vi "Parse.vi"(8 "Error In":errorcluster, 11 "object in":refnum<class "2024_2.lvclass">) -> (0 "Error Out":errorcluster, 3 "object out":refnum<class "2024_2.lvclass">)   [LabVIEW 2023, in "2024_2.lvclass"]
uses:
  2024_2.lvclass
  2024_2.lvclass/2024_2.ctl
  <vilib>/Utility/error.llb/Trim Whitespace One-Sided.vi
  <userlib>/_OpenG.lib/string/string.llb/openg_string.lvlib
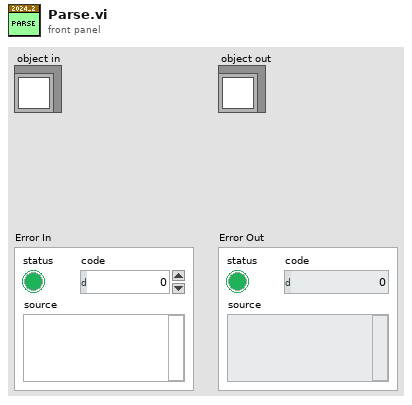
[diagram p1: front panel]
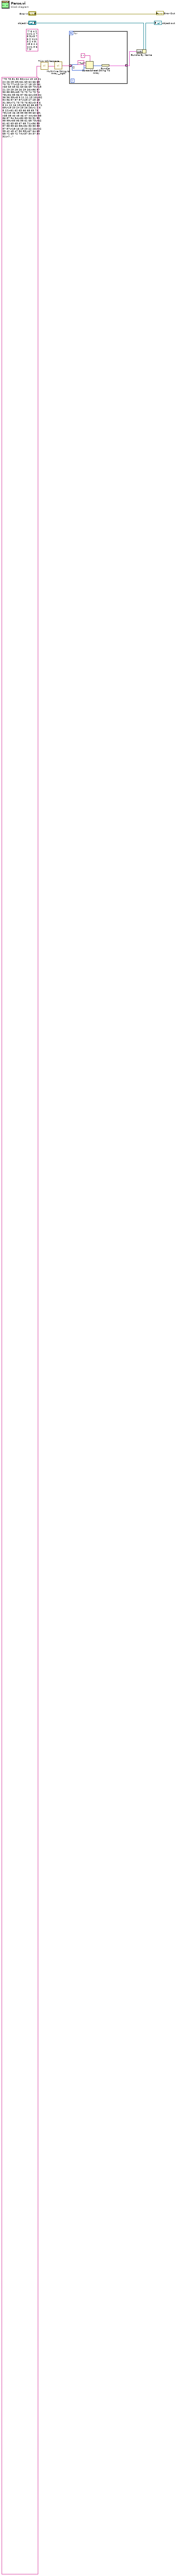
[diagram p0: block diagram]
diagram:
  (unwired) "7 6 4 2 1\n1 2 7 8 9\n9 7 6 2 1\n1 3 2 4 5\n8 6 4 4 1\n1 3 6 7 9" ("PuzzleInput")
  n1 = call <vilib>:"Trim Whitespace.vi"("string"="75 78 81 82 80\n14 15 18 21 24 26 28 28\n61 63 64 66 68 70 73 77\n13 14 17 18 19 26\n60 63 65 62 63 66 69 70\n18 21 23 25 28 26 29 26\n86 87 90 88 88\n69 70 73 74 73 74 78\n54 55 56 57 56 62\n33 34 36 36 39\n8 9 11 11 13 10\n52 54 56 57 57 57\n25 27 28 28 31 35\n71 73 73 76 82\n3 5 6 8 11 12 16 19\n59 62 66 69 71 69\n19 20 24 25 26 26\n1 2 6 8 12\n61 62 63 66 68 69 73 78\n43 46 48 55 58 59 60 63\n35 38 40 45 46 47 44\n84 85 86 87 94 94\n80 83 90 91 93 95 99\n53 56 58 61 68 73\n62 61 62 63 65 67 68 71\n56 55 57 58 59 60 58\n52 50 53 55 57 57\n18 16 19 20 22 26\n42 39 42 45 47 50 55\n67 64 65 68 71 69 72 74\n37 34 37 34 31\n75 72 74 73 75 77 77\n90 88 90 91 90 91 95\n72 70 72 69 70 76\n71 70 71 71 73\n83 80 80 81 80\n68 66 69 72 72 75 75\n45 44 45 48 48 50 54\n64 62 65 65 72\n39 37 39 43 46 48 51 52\n28 27 31 33 32\n25 22 26 29 29\n72 71 72 75 79 82 86\n70 68 71 75 76 78 81 88\n89 87 89 90 96 97\n8 7 9 14 17 16\n31 29 30 37 40 43 45 45\n44 41 43 50 52 53 57\n4 1 2 9 15\n6 6 9 11 12 13 16\n36 36 37 40 43 45 47 46\n88 88 89 91 94 94\n13 13 16 19 21 22 26\n17 17 19 20 21 24 26 31\n21 21 22 21 24\n73 73 71 72 74 77 80 79\n31 31 33 34 37 36 36\n21 21 20 23 27\n31 31 29 31 37\n55 55 58 60 60 63 64\n28 28 31 31 29\n69 69 70 73 74 74 74\n12 12 15 17 18 18 19 23\n5 5 5 6 13\n61 61 63 67 68\n37 37 39 42 43 47 46\n76 76 79 82 86 86\n43 43 47 50 53 55 56 60\n51 51 52 55 59 60 67\n75 75 78 81 88 90 92\n53 53 55 57 59 61 68 67\n86 86 87 88 94 94\n60 60 62 64 67 74 78\n71 71 74 81 83 86 93\n22 26 29 30 31 32 34 36\n47 51 52 55 57 55\n39 43 45 46 46\n72 76 79 82 83 87\n38 42 44 47 50 51 52 57\n79 83 81 84 86\n3 7 4 7 8 11 12 10\n44 48 50 52 51 54 54\n83 87 90 92 89 93\n68 72 73 76 74 81\n24 28 31 31 32 34 37\n58 62 62 63 65 66 64\n28 32 32 35 35\n40 44 45 45 47 50 51 55\n31 35 36 37 39 42 42 49\n17 21 24 26 30 32 33 35\n67 71 73 74 78 81 78\n79 83 85 89 92 92\n37 41 44 45 46 50 54\n72 76 79 81 85 88 89 96\n46 50 57 58 59 62 65\n66 70 75 76 77 75\n16 20 26 29 29\n32 36 41 42 44 46 50\n61 65 66 68 75 78 80 85\n14 19 20 22 25 27 29 31\n16 22 24 26 24\n5 12 14 17 18 19 22 22\n16 22 24 27 29 30 32 36\n37 43 46 49 52 53 60\n10 16 13 15 16 19\n67 73 76 75 73\n1 7 9 10 8 8\n37 42 41 44 46 48 50 54\n62 67 66 68 74\n41 48 51 51 53\n53 59 62 63 63 66 65\n66 73 73 76 76\n49 55 55 56 60\n43 50 50 52 54 57 64\n9 15 18 22 25\n10 15 19 20 22 19\n34 41 42 46 47 48 51 51\n24 30 34 36 37 40 43 47\n39 46 50 51 57\n11 18 21 23 26 32 34\n62 67 70 77 75\n80 86 91 92 93 93\n65 72 73 80 83 87\n39 46 48 54 59\n79 76 74 73 70 73\n13 12 11 9 9\n53 51 49 47 43\n59 58 55 52 50 47 46 39\n8 6 9 6 5 4 3 1\n26 23 25 23 22 24\n62 61 64 61 60 58 57 57\n59 58 59 57 55 51\n28 26 23 24 21 20 15\n80 77 76 76 74 73\n35 34 31 30 30 31\n7 6 5 5 5\n99 96 93 92 92 89 85\n74 73 72 72 71 70 69 62\n28 27 25 21 20\n40 38 35 32 29 25 24 25\n96 93 90 88 87 83 80 80\n32 29 25 22 18\n39 36 33 29 27 24 18\n44 41 38 37 31 30\n62 61 54 51 54\n83 81 74 72 71 68 68\n33 30 28 27 24 18 16 12\n91 89 88 87 82 80 78 73\n31 34 33 32 31 29 26 24\n16 17 15 14 17\n51 54 51 49 46 46\n91 92 89 86 85 81\n36 39 36 33 32 27\n12 14 16 14 13 10 8\n87 90 87 84 82 80 83 86\n47 48 47 46 44 43 46 46\n86 87 88 87 85 82 79 75\n69 70 69 66 65 64 65 58\n57 60 59 59 57\n83 85 84 84 87\n84 85 83 80 79 78 78 78\n93 94 92 89 89 85\n41 42 40 37 37 35 33 26\n32 34 30 27 25 23\n42 44 40 38 37 34 31 33\n72 75 74 71 67 64 62 62\n87 88 86 85 81 77\n43 46 43 39 38 37 31\n82 84 82 81 74 72\n35 37 32 31 30 32\n58 60 59 54 54\n90 92 89 84 82 78\n87 89 88 83 81 80 78 73\n30 30 27 26 25\n44 44 43 40 39 37 35 36\n61 61 59 58 55 55\n25 25 24 21 17\n85 85 84 82 79 78 73\n77 77 75 77 75 72\n78 78 76 79 80\n42 42 40 38 40 38 37 37\n59 59 58 59 58 54\n58 58 56 55 53 52 55 49\n75 75 74 74 72 71 68 66\n72 72 72 69 68 67 68\n39 39 36 36 33 33\n32 32 32 29 27 26 24 20\n92 92 91 90 89 88 88 83\n51 51 50 49 48 44 43\n36 36 35 34 32 28 26 29\n81 81 78 76 73 69 69\n18 18 14 12 9 8 6 2\n65 65 61 59 57 54 47\n90 90 83 82 81\n90 90 83 81 79 77 74 77\n46 46 43 37 36 33 33\n22 22 20 17 11 8 4\n78 78 72 71 69 66 61\n58 54 52 50 48\n51 47 45 44 42 41 43\n39 35 32 29 29\n50 46 43 40 37 36 35 31\n35 31 29 28 27 26 24 18\n95 91 88 85 88 85 82\n96 92 89 87 86 84 85 86\n68 64 61 64 63 63\n40 36 35 37 33\n46 42 44 43 41 38 33\n17 13 11 10 7 7 5 3\n78 74 71 69 68 68 70\n58 54 51 51 50 48 48\n49 45 43 42 42 40 36\n42 38 38 35 34 29\n25 21 20 17 16 12 10\n98 94 90 87 90\n75 71 67 64 61 58 58\n77 73 70 68 66 62 58\n74 70 68 64 62 59 53\n69 65 59 56 55 53\n86 82 79 76 74 69 70\n57 53 50 44 43 40 40\n28 24 18 15 14 11 7\n76 72 71 69 64 61 55\n92 86 85 83 80 78 75\n31 24 23 21 19 17 20\n66 61 58 57 54 54\n92 86 85 82 81 80 76\n37 31 30 28 25 22 17\n72 67 69 68 65 63\n15 8 6 9 11\n17 11 14 12 11 9 6 6\n27 22 19 20 17 15 14 10\n62 57 54 52 50 51 44\n86 79 77 77 75 74\n51 44 44 42 43\n42 36 36 35 34 33 30 30\n39 32 30 29 27 27 25 21\n91 84 84 81 75\n40 35 31 28 26 23 21 18\n73 67 66 64 61 57 60\n39 33 29 27 25 23 23\n50 43 40 39 36 35 31 27\n60 54 53 52 48 45 42 37\n90 84 83 82 75 74 72\n82 76 73 70 69 62 59 62\n58 51 48 45 38 36 36\n96 91 90 85 81\n53 48 45 44 43 37 36 30\n47 48 50 53 52\n49 50 53 54 56 57 57\n43 46 47 49 52 56\n84 85 86 87 88 91 96\n41 42 45 47 44 46\n58 59 60 58 59 60 57\n88 91 94 92 95 96 96\n42 44 41 44 48\n36 38 37 40 47\n55 58 60 60 63\n6 7 9 9 7\n33 35 38 41 42 43 43 43\n4 6 6 9 12 16\n9 10 12 12 13 16 23\n74 75 79 82 85 88 91\n71 73 76 80 83 80\n70 71 75 77 79 79\n36 38 41 43 47 51\n63 66 69 70 71 72 76 81\n4 6 8 9 12 14 20 22\n32 35 37 44 47 50 52 51\n7 10 16 18 19 21 21\n24 26 32 33 34 36 38 42\n43 44 51 53 59\n62 59 61 63 65 67 70\n28 25 27 28 30 33 34 33\n46 45 47 49 50 51 51\n7 6 9 10 12 16\n29 27 29 32 38\n46 45 47 45 46\n4 2 4 5 8 9 6 5\n9 8 5 8 10 10\n80 78 75 76 80\n51 50 51 52 53 52 55 61\n26 24 25 27 27 28\n87 86 88 90 91 91 94 91\n30 29 29 31 33 34 35 35\n31 30 30 33 36 40\n29 27 27 30 32 35 36 41\n75 72 75 77 81 84\n22 20 22 26 25\n74 71 75 76 76\n55 53 56 60 61 65\n49 48 52 53 59\n8 7 8 15 18 20\n4 2 4 10 13 10\n31 28 35 38 39 41 41\n76 75 80 81 83 87\n54 53 59 60 65\n45 45 47 50 52 54 57 58\n31 31 34 36 39 41 43 40\n70 70 72 75 75\n38 38 40 43 45 48 52\n51 51 52 54 60\n69 69 70 69 70\n59 59 61 64 63 65 63\n32 32 34 32 32\n71 71 70 73 75 79\n71 71 68 69 76\n16 16 19 19 21 23 24\n58 58 60 60 58\n13 13 16 19 19 19\n53 53 55 55 59\n84 84 87 88 88 89 95\n8 8 12 13 16\n50 50 52 56 54\n17 17 20 22 26 29 29\n9 9 11 12 16 19 23\n23 23 25 29 30 33 35 42\n21 21 22 29 30\n51 51 52 54 55 61 58\n21 21 24 31 33 34 35 35\n75 75 80 82 86\n42 42 45 51 56\n21 25 28 31 33 36\n35 39 40 41 42 41\n1 5 7 10 12 13 13\n77 81 82 83 86 88 92\n40 44 47 50 56\n49 53 51 52 53 55 56\n63 67 68 71 69 66\n79 83 82 83 83\n89 93 96 97 95 99\n71 75 76 73 79\n62 66 66 68 71\n18 22 22 25 26 27 28 27\n13 17 17 19 19\n54 58 58 61 65\n43 47 48 50 51 51 56\n86 90 92 96 98\n51 55 56 60 61 59\n49 53 54 56 59 63 63\n34 38 39 41 43 46 50 54\n82 86 90 91 96\n40 44 46 48 53 56\n1 5 7 12 10\n76 80 86 89 92 94 97 97\n42 46 48 53 56 58 62\n60 64 66 69 71 78 80 86\n61 68 71 74 76 77 78\n64 70 72 75 78 76\n78 83 85 87 87\n50 55 56 57 61\n80 86 89 92 99\n51 56 59 62 64 62 64\n24 30 31 29 30 32 29\n84 89 91 92 89 89\n49 54 55 58 59 62 60 64\n16 23 22 24 25 28 34\n23 28 28 31 34 37 40 42\n8 14 17 17 20 19\n46 52 52 53 53\n52 59 59 61 64 68\n29 36 38 40 42 42 43 48\n62 68 71 74 77 79 83 84\n75 80 81 82 86 83\n72 78 80 84 86 88 91 91\n45 50 54 57 58 61 65\n14 21 24 27 30 31 35 40\n16 21 28 31 34\n28 33 38 39 38\n48 54 60 61 61\n25 31 33 34 41 45\n11 17 20 25 28 33\n30 27 26 24 22 24\n32 30 28 26 24 22 22\n46 44 43 41 39 35\n65 62 60 59 57 52\n22 20 17 14 11 13 10 8\n78 76 73 76 75 73 72 75\n47 44 43 40 42 41 40 40\n70 67 69 67 63\n11 9 7 8 3\n35 34 31 29 29 27 26 24\n88 85 85 82 84\n78 76 76 75 74 73 73\n76 75 72 72 70 69 65\n32 29 27 27 26 19\n49 47 43 41 38 36\n67 65 64 60 59 58 55 57\n83 81 80 77 73 73\n22 21 17 16 14 12 8\n29 28 24 22 21 14\n90 88 83 80 77 74\n58 56 55 48 45 48\n12 11 8 3 2 2\n94 91 86 84 82 78\n64 61 54 51 50 47 45 38\n21 23 22 19 17 16\n62 63 62 60 59 56 58\n46 49 46 44 42 41 41\n83 86 83 81 80 78 74\n52 54 51 50 48 45 42 37\n49 52 50 51 50\n50 52 50 53 56\n39 40 43 41 40 39 37 37\n71 72 70 68 69 66 62\n42 45 42 39 40 33\n45 46 43 40 37 37 35\n80 82 82 80 79 78 80\n86 89 88 87 87 85 82 82\n22 23 20 20 19 15\n77 78 77 74 74 72 65\n24 27 23 22 20\n53 55 53 51 47 49\n17 20 16 15 12 10 7 7\n87 89 88 87 86 85 81 77\n28 30 26 23 21 16\n57 58 55 54 48 45\n78 80 79 72 70 73\n75 77 72 69 69\n29 31 25 22 19 16 12\n67 68 65 60 54\n20 20 17 15 12 9\n33 33 32 29 27 28\n87 87 84 82 79 78 78\n13 13 12 10 9 5\n79 79 78 76 75 70\n97 97 98 97 94\n75 75 74 73 72 71 72 75\n65 65 66 65 63 63\n66 66 69 66 62\n12 12 10 7 9 3\n18 18 17 17 16 13 12 10\n25 25 25 23 24\n27 27 25 22 20 20 19 19\n85 85 85 84 82 78\n26 26 26 25 24 22 21 14\n76 76 73 70 66 64 62 60\n54 54 50 48 46 48\n14 14 13 9 9\n61 61 59 55 52 51 47\n78 78 76 72 67\n38 38 33 32 29\n57 57 51 48 46 47\n41 41 36 33 30 27 27\n74 74 68 67 63\n69 69 62 60 58 52\n25 21 19 16 14 11\n39 35 33 30 28 25 22 25\n58 54 52 51 50 49 49\n31 27 25 24 21 19 17 13\n83 79 77 76 75 74 71 64\n38 34 37 35 34\n50 46 43 42 45 46\n78 74 77 76 73 73\n14 10 9 10 9 5\n33 29 31 30 24\n41 37 37 35 32\n62 58 57 55 55 58\n17 13 11 9 6 6 4 4\n25 21 19 17 15 15 11\n60 56 56 53 48\n53 49 45 42 40\n34 30 28 26 25 21 20 22\n99 95 94 90 89 88 85 85\n43 39 35 33 31 27\n75 71 69 67 63 57\n59 55 54 47 44\n48 44 37 34 36\n42 38 33 30 27 27\n63 59 54 53 50 47 43\n71 67 66 60 57 54 48\n55 48 46 44 41\n56 49 48 45 42 45\n89 84 82 79 77 74 74\n51 44 41 38 35 33 29\n88 82 80 77 70\n81 75 72 75 72\n58 52 51 48 45 46 43 44\n78 72 71 68 70 68 65 65\n52 47 50 48 47 44 43 39\n18 11 14 11 8 7 6 1\n78 72 70 70 68 67 66\n72 65 63 63 61 63\n28 21 21 19 16 13 11 11\n89 82 82 81 77\n50 44 44 43 40 38 33\n70 65 62 59 58 54 51 48\n29 22 21 19 16 12 15\n82 76 74 70 67 64 64\n20 14 11 7 3\n42 36 35 31 30 27 24 19\n64 58 56 54 51 45 42 41\n29 24 22 21 16 14 11 13\n62 57 52 50 50\n65 59 52 49 46 44 42 38\n76 71 66 64 58\n41 47 50 53 52\n26 20 17 15 15\n76 77 84 86 87 87\n16 13 13 11 5\n63 61 59 57 54 51 50 46\n69 69 63 62 59\n94 92 91 92 89 86 83 86\n83 87 90 92 94 98 98\n69 69 70 71 75\n81 78 81 81 86\n82 76 75 72 68 67 66 66\n86 84 81 84 79\n10 9 10 12 13 15 16\n49 53 50 53 55 52\n84 87 89 90 89 90 94\n24 24 22 24 21 20 22\n77 79 72 70 68 71\n33 35 33 31 28 23 17\n35 33 31 26 25 23 22 22\n70 74 77 77 78 81 84 84\n72 69 67 64 63 66 63\n36 39 40 40 42 45 42\n20 16 16 15 13\n54 47 46 41 41\n64 63 62 60 58 60 56\n33 26 28 25 22 19 18 12\n2 6 9 12 12 13 11\n42 45 49 52 54 51\n84 78 78 75 74 72 72\n84 84 83 81 80 77 73 68\n71 71 75 76 83\n67 67 64 58 56 52\n52 57 54 55 56 57 59\n96 94 92 91 87 80\n74 69 67 66 62 64\n60 60 62 63 62\n85 81 79 79 79\n53 57 59 60 62 65\n72 74 75 76 77 78 82\n19 15 13 9 7\n60 53 50 49 47 45 40\n41 37 36 33 30 26 22\n43 45 42 40 37 31\n19 26 29 31 33 37\n49 42 41 40 39 40\n46 46 49 47 47\n71 66 63 60 55 52 49 50\n24 28 29 30 31 37 40 39\n23 23 22 21 19 18 15 9\n48 48 51 51 51\n39 39 38 34 30\n37 37 39 42 45 48 54 51\n30 28 25 23 21 18 16 17\n30 31 34 39 37\n46 51 52 54 54 55 57\n94 94 93 94 90\n41 45 46 47 50 56 57 57\n65 66 64 60 61\n28 27 28 35 41\n83 83 83 80 80\n81 77 74 71 71 67\n86 83 82 81 79 76 71\n79 72 69 65 64 61\n86 88 87 86 85 82 82 78\n32 33 33 34 37 40 43\n5 9 11 13 16 19 18\n16 13 15 18 15\n47 43 40 37 35 31\n46 39 37 37 35 31\n3 3 6 6 5\n48 52 53 55 56 59 59 66\n43 44 44 47 49 55\n54 59 62 69 70\n40 40 38 36 34 31 27 24\n98 91 91 88 85 88\n20 20 21 25 26 27 29 29\n88 82 84 81 81\n85 85 82 80 79 78 76\n79 81 77 74 72 71 70\n38 34 30 28 25 18\n88 85 83 80 77 77 77\n66 66 65 62 62 60 56\n31 34 32 30 29 27\n26 24 27 26 26\n94 94 93 86 85 84 83 85\n28 27 28 32 34 35 37 37\n97 95 95 94 92 93\n62 62 64 62 63 66 68 72\n70 70 67 64 61 59 59\n76 73 69 67 67\n42 42 38 37 37\n25 29 32 33 36 40 42 40\n49 52 52 55 56 57 61\n85 83 84 87 93\n46 50 56 58 60 61\n22 18 15 11 8 5 8\n68 64 63 63 66\n10 10 11 13 16 19 21\n18 14 11 8 6 4 3 1\n54 55 54 55 52 52\n46 46 48 50 47 50 52\n94 90 89 88 85 83 84\n79 86 87 88 91 95 92\n78 78 80 84 82\n11 11 12 15 16 17 20 20\n16 22 20 23 24 26 33\n51 50 47 44 42 40 38 38\n53 46 45 44 42 39\n67 67 66 65 59 54\n66 71 71 74 75 77 79 79\n36 32 31 28 28\n17 14 21 23 21\n86 83 81 77 75\n62 55 50 49 45\n19 25 26 27 30 31 28 28\n34 38 41 47 48 49 51 55\n51 51 49 47 46 42\n78 78 76 76 75 74 73 75\n81 85 86 89 93 98\n76 72 73 72 70\n15 17 16 13 15 11\n44 46 49 56 58 59\n43 43 45 45 48 51 53 60\n88 84 83 80 78 79 82\n37 33 30 29 28 30 27 20\n45 51 54 56 59 61 63 63\n45 44 47 47 48 46\n52 46 44 40 33\n27 33 36 39 45 47 50 55\n76 78 79 84 88\n14 13 12 11 7 4 5\n59 64 68 69 70 71 71\n74 67 70 68 66 64 62\n76 76 74 74 73 70 64\n31 35 35 36 39 40 43 45\n94 92 93 91 93 94 96 99\n11 11 10 11 12 15 15\n25 22 25 26 26 28 28\n33 35 35 32 30 28 27 29\n50 52 50 47 43 43\n73 77 80 77 80 81 83 87\n78 75 78 81 84 86 83 89\n39 41 39 42 44 42\n42 40 40 39 35\n73 70 69 64 61 57\n99 92 91 88 81 74\n95 96 89 86 85 81\n1 1 1 4 7 11\n36 37 30 27 26 24 21\n23 20 16 13 11 7\n54 57 56 55 56 58\n92 88 86 85 85 82 80 74\n20 23 21 21 20 17 15 9\n11 15 16 17 17 20 21 25\n36 40 39 42 44 51\n36 32 31 30 25 23 19\n80 84 86 92 97\n19 20 18 14 10\n4 3 6 8 9 13 16\n84 84 88 91 95\n26 26 24 21 18 15 18\n99 92 89 86 88 85 87\n68 66 68 71 73 76 80 86\n23 22 27 29 33\n65 68 68 67 66 65\n46 50 52 55 59 60 62 65\n45 51 52 53 56 56 58 55\n20 26 27 29 31 34 36 41\n15 15 16 18 16 21\n62 58 56 52 49 48 47 47\n8 11 14 17 19 22 20\n54 55 57 59 65 68 70 77\n60 56 54 51 50 45 42 36\n57 54 58 60 64\n32 36 39 42 43 46 49 55\n46 45 48 51 52 59 61\n30 26 19 18 17 16 14 14\n81 84 81 84 87 90 91\n84 85 84 81 83 77\n27 20 13 10 7 6 3\n63 59 56 54 51 45\n14 14 11 13 8\n53 49 46 49 46 44 44\n61 64 67 68 69 72 74 77\n58 60 61 64 65 68 71\n61 63 65 68 71 74 76\n18 21 24 27 30 32\n15 17 18 21 22 24 26\n40 41 44 46 48 49 51\n35 37 39 41 44 45\n9 12 13 15 17 20\n32 34 36 38 40 43\n60 58 57 55 52 49\n68 67 65 62 60 57 55 53\n34 35 36 39 42 45 47 48\n22 21 20 18 16 13 10 9\n76 77 79 81 83\n81 82 85 86 89 92 95\n24 27 28 30 31 34 37 40\n2 5 8 10 13 15 18\n76 79 81 84 87 88\n41 40 39 37 36 34 33 32\n29 27 25 22 21 18\n83 81 78 77 74 73 72\n97 94 92 90 89\n35 37 40 42 45 48\n33 32 30 29 27 25\n18 17 16 15 14 11 10\n67 69 70 71 73 76 77 80\n44 43 41 40 37 36\n68 65 63 62 61 59\n87 86 83 82 80 78\n41 38 37 34 31 29\n5 7 8 11 13 14\n59 61 62 65 66\n20 21 24 26 28 31 32 33\n33 36 38 39 41 42 44\n42 41 39 37 34 33 31\n18 21 23 26 29 32 33\n88 87 85 82 79\n60 61 62 65 68\n82 80 77 76 73\n20 18 15 14 11 9\n84 82 79 77 74 73 72 70\n66 63 62 61 58 56 53\n44 43 41 39 37\n82 79 78 75 73 72 69\n76 77 78 81 82 84\n8 11 13 14 16 18\n17 20 22 25 27 30 31 32\n74 72 70 67 65 63 60 57\n14 13 11 9 8 7 5\n59 61 63 66 67 70\n81 83 84 85 88 91\n42 41 39 37 34 33\n36 39 40 41 42\n56 55 52 49 46 43 41 38\n74 73 72 69 66 63 60\n80 81 82 85 87\n56 57 59 60 61\n9 8 7 6 3 2\n22 19 18 17 16\n36 39 41 44 46 48 49\n4 7 9 12 14 17\n46 44 43 41 38 36 33 32\n86 84 82 81 78\n61 64 65 66 67 69\n45 47 49 50 52 54\n24 22 20 19 18 17\n23 25 27 28 29 31 32\n36 33 31 28 26\n7 9 12 14 16\n8 11 14 17 18 19 20\n86 88 90 92 95 97 98\n74 75 78 81 82\n68 66 65 62 59 56\n57 58 61 62 63\n35 37 39 41 43 45 46 48\n87 85 84 81 78 75 72\n59 58 57 54 51\n67 68 71 72 74\n12 13 16 19 20\n39 42 45 47 50 53 54 55\n78 76 74 73 72 71 70\n16 17 19 21 22 23 25 27\n26 28 29 31 33\n50 51 54 55 58 60 61 63\n81 84 85 88 90 92 94\n99 97 95 93 90 89 86\n26 29 30 31 33\n49 46 43 42 39 38 37 35\n49 48 46 45 43 41 38\n22 20 18 16 14 11 9\n13 15 17 19 22 23 26 28\n70 73 75 78 79\n82 81 79 76 73 70 68 66\n35 34 33 31 29 26\n16 14 13 12 9 8 5 3\n73 74 76 77 79 82 85 88\n61 64 66 69 72 75\n89 90 93 95 96\n84 81 80 77 75 72 69\n10 9 8 7 5 3 1\n95 94 92 91 88 87 86\n51 52 53 56 57\n98 97 95 92 89 88 87 86\n74 72 71 68 65\n61 59 58 56 53\n46 49 50 51 53 55 57 59\n86 83 80 79 76\n44 42 41 38 37\n53 54 56 57 60 63 65 68\n62 63 64 65 67\n94 91 88 87 86\n47 44 42 39 37 34\n42 44 45 48 49 52\n44 42 40 38 35 33 31 28\n55 52 50 47 46 44\n80 79 76 75 73 71 68\n51 49 48 46 44\n13 16 19 21 22\n42 40 39 38 35 34 31 29\n63 62 60 57 55 52\n52 49 46 44 43 41 38\n16 13 11 10 8 7 6\n57 58 60 62 65 68 69 71\n23 22 19 16 14 11 9\n56 55 52 51 50 49\n15 13 11 8 7\n70 68 65 63 62 59\n76 79 80 81 83 86 89\n74 71 69 68 66 63 61 60\n18 16 13 10 7 6 3 1\n49 47 44 42 41 39 38 35\n80 78 77 76 74 73\n91 94 95 97 99\n70 69 68 66 64\n58 60 61 62 63 66\n62 63 66 69 70 72 73\n50 51 53 54 57 59\n34 32 29 26 25\n11 9 8 5 2\n42 39 36 35 33 31 28\n56 59 61 62 65 67\n80 77 76 73 70 69\n42 40 38 35 32\n61 63 64 67 70\n90 89 87 84 83 81 80 77\n36 33 30 29 26 25 22 21\n60 58 56 54 53 50 49\n87 89 91 93 96 98\n49 52 53 56 59\n35 38 40 43 45 46 47 50\n41 44 45 48 49\n75 72 71 69 68 67 64\n36 34 31 30 28 26 25 23\n18 15 14 12 11\n42 39 38 37 35\n38 40 41 42 44 47\n16 14 11 8 7\n31 30 27 26 25\n66 68 70 71 72 74\n58 57 54 51 49 47 45 44\n31 34 36 39 41 42\n51 49 48 47 46 43 41 39\n43 44 45 47 48 50\n90 89 88 87 84 82 79\n21 24 26 28 30 31\n53 50 47 45 42 41\n27 24 22 21 19\n25 28 29 32 33 34\n12 13 15 18 20 21 23 26\n75 72 71 70 68 67 64\n14 11 9 7 4 2\n31 32 34 36 39 41 43 46\n55 57 58 59 61 64\n45 47 50 51 53\n53 51 49 48 45 43 41 40\n28 30 31 34 35 36 39\n55 52 51 50 48 47 45\n5 8 9 11 13 16 17 20\n66 68 69 72 75 78\n62 65 67 70 73\n45 47 50 51 52 55\n27 29 31 32 34\n90 89 86 85 84 81 78\n66 63 61 59 58 57\n44 42 41 38 35\n80 83 84 86 87 90 92\n93 90 87 86 85\n64 66 67 68 71 74 77 80\n52 53 54 56 58 59 61 62\n75 74 73 72 70 68\n93 91 88 87 86 84 81 80\n10 11 13 16 19\n81 80 78 75 72 69 66 64\n50 48 45 42 41 38 35 34\n66 69 72 75 78 80 82 85\n75 72 70 67 64\n33 31 30 28 26 25 23\n51 54 57 59 62 64 65\n39 42 44 45 47 50\n24 25 27 29 31\n18 15 14 12 9 6 5 4\n15 14 13 10 8 5 3 1\n13 14 17 19 20 23 25 28\n45 42 41 38 37\n49 47 45 44 41 38 36 34\n26 29 32 35 37\n24 26 27 29 31\n68 70 72 73 76 79 82\n60 59 57 54 52 49 46 43\n58 59 60 62 65 66\n12 14 15 18 19 21\n85 88 89 90 93 96\n22 23 24 27 28 29 31\n38 41 44 47 49 52\n52 49 47 45 42 40 39\n77 78 79 80 81\n32 35 36 38 40 42 43 44\n70 72 73 75 78\n36 37 38 41 43 46\n40 42 45 46 48 51\n23 22 20 19 17 16 15\n93 91 88 87 85\n36 35 32 31 28 26\n61 62 64 67 68 70 73\n38 35 32 30 28\n6 9 12 13 16 18 19\n48 51 52 53 55 57 58\n16 14 12 9 6 5 4 2\n49 48 47 44 41 39 37 36\n70 67 65 63 62 59 57 56\n46 48 50 51 54\n83 80 77 76 74 72 70 68\n58 55 53 51 48 46 45 42\n37 40 43 45 46\n6 8 10 13 15 16 18\n32 33 36 37 39\n24 21 19 18 16 15 12 9\n54 52 50 47 45\n6 7 9 11 12 14 16 17\n85 84 83 81 79\n60 63 65 68 69 71 74 75\n71 73 76 78 81 83 86 87\n17 15 14 12 9\n35 36 39 40 41\n53 56 57 60 61 63\n66 69 72 74 77 79\n2 3 4 6 8 10\n15 12 9 8 5 3\n39 40 41 44 46 47 50\n77 75 74 71 69 66\n78 79 81 82 83 86\n60 58 57 55 54 51 48 45\n38 39 40 41 44\n47 46 44 43 41 40 39 36\n70 68 67 64 62 59 56 54\n19 22 24 27 30 33 35 38\n57 54 53 50 47\n16 18 19 22 24 27\n62 60 57 54 53 51 50\n6 7 8 11 14 15\n30 32 35 38 39 42\n23 22 19 17 15\n70 73 76 78 80\n87 84 83 80 78\n81 83 85 87 88 90 91 92\n34 33 31 28 25 24\n79 77 75 73 70 67 64 61\n20 21 24 25 26 29 32\n58 61 63 65 68 70 72\n17 20 23 24 27 30\n73 76 79 80 83 86 88 90\n50 52 54 57 60\n15 13 11 10 8 5 3 2\n91 89 88 86 83 81\n81 84 86 88 90 92\n82 85 88 91 94\n28 30 32 35 38 39 40 42\n88 86 83 80 77 76 74 71\n43 41 39 37 34\n34 36 37 38 39\n67 65 63 61 60 57 56\n50 47 44 42 41 39\n42 44 45 47 49 52 55 58\n23 24 25 26 27 29 30\n80 78 76 75 72 69 66 65\n33 36 37 40 41 44 46\n19 22 25 26 28 29\n19 20 23 24 26\n86 87 88 90 91 93 94 96\n75 76 77 78 80\n10 13 16 19 20 22 23 26\n11 13 14 15 18 20\n78 81 82 83 86 87\n81 82 84 85 86 87\n67 68 70 72 75\n17 16 13 11 9 7 4\n90 91 94 95 96 99\n84 85 87 88 89 92\n90 89 88 87 84 81\n22 24 27 30 32 35 36 37\n55 52 50 47 44\n99 97 94 92 91 89\n25 22 21 19 18 17\n45 44 42 41 39 36 35 34\n48 46 43 41 40 37\n29 31 34 37 39\n54 53 51 49 47 46 45\n13 10 9 7 5 3\n61 60 58 57 55 54 52 49\n54 53 51 48 46 44 41 40\n22 21 20 17 15 14 11 10\n46 45 44 42 39 37 35 32\n80 82 84 85 88\n42 40 38 36 35 33 32\n49 50 52 54 57 60\n62 65 68 71 72 74 77 80\n69 66 63 62 61 59 58\n42 41 38 36 33 30\n55 54 51 50 47\n35 33 31 30 28 27 26\n55 58 60 63 65" ("PuzzleInput")) -> ("trimmed string"=w4:string)  [unwired: 1 in]
  n2 = call <userlib>:"Multi-line String to Array__ogtk.vi"("string"=w4) -> ("lines"=w3:string[])
  n3 = for {
    tunnel: w3 -> [w13] mode=indexing
    tunnel: [w8] -> w2 mode=indexing
    n4 = Spreadsheet String To Array(delimiter (Tab)=" ", format string="%d", spreadsheet string=w13, array type (2D Dbl)=i32[] []) -> (array=w9:i32[])
    n5 = Bundle("array type (2D Dbl)"=w9) -> (w8:cluster{"array type (2D Dbl)":i32[]})  [unwired: 1 in]
  }
  n6 = Bundle By Name(cluster="object in", "List"=w2) -> (→"object out":refnum<class "2024_2.lvclass">)
  "Error Out" <- "Error In"
